vi "WristStartPose.vi"(8 "error in (no error)":errorcluster) -> (0 "WristStartPose":dbl, 3 "error out":errorcluster)   [LabVIEW 2023]
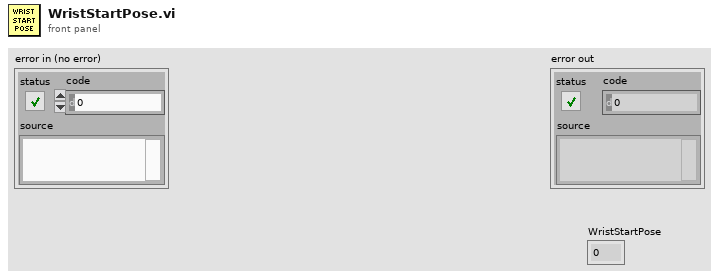
[diagram p1: front panel]
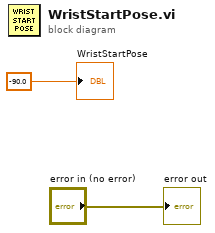
[diagram p0: block diagram]
diagram:
  "WristStartPose" <- -90.0 ("Numeric")
  "error out" <- "error in (no error)"
